vi "SUMMER SUNDAY BYTE.vi"() -> ()   [LabVIEW 2009]
uses:
  <vilib>/ULx/Create Channel.llb/ULx Create Channel (AI-Voltage-Basic).vi
  <vilib>/ULx/Read.llb/ULx Read (Analog DBL 1Chan 1Samp).vi
panel:
  in  "BitValue":bool
  out "POWER":bool
  out "data":dbl format="%_6g"
  out "xray":bool caption="BitValue"
  out "ENERGY LEVEL":dbl(knob) scale=0.0..15.0
  out "x*y":dbl
  out "Beam Pot":dbl format="%_6g"
  out "READY 2":bool
  out "DUMP":bool
  out "POWER":bool
  out "?":bool
  out "?":bool
  out "?":bool
  out "?":bool
  out "?":bool
  out "?":bool
  out "?":bool
  out "?":bool
  out "?":bool
  out "?":bool
  out "OPEN":bool
  out "CLOSED":bool
  in  "READY":bool
  out "FAULT":bool
  out "MAGNET FORCE":dbl(slide) scale=0.0..10.0
  out "READY":bool
  out "TEMPERATURE":dbl(slide) scale=0.0..10.0
  in  "stop":bool
  out "?":bool
  out "?":bool
  out "?":bool
  out "?":bool
  in  "FAULT":bool
  out "POWER":bool
  out "FLOW IN GPM":dbl(knob) scale=0.0..15.0
  # "USERS LAB AREA"
  # "BEAM STATUS"
  # "ROOM"
  # "XRAY"
  # "PUMP STATION"
  # "MAGNET STATUS"
  # "ORBIT"
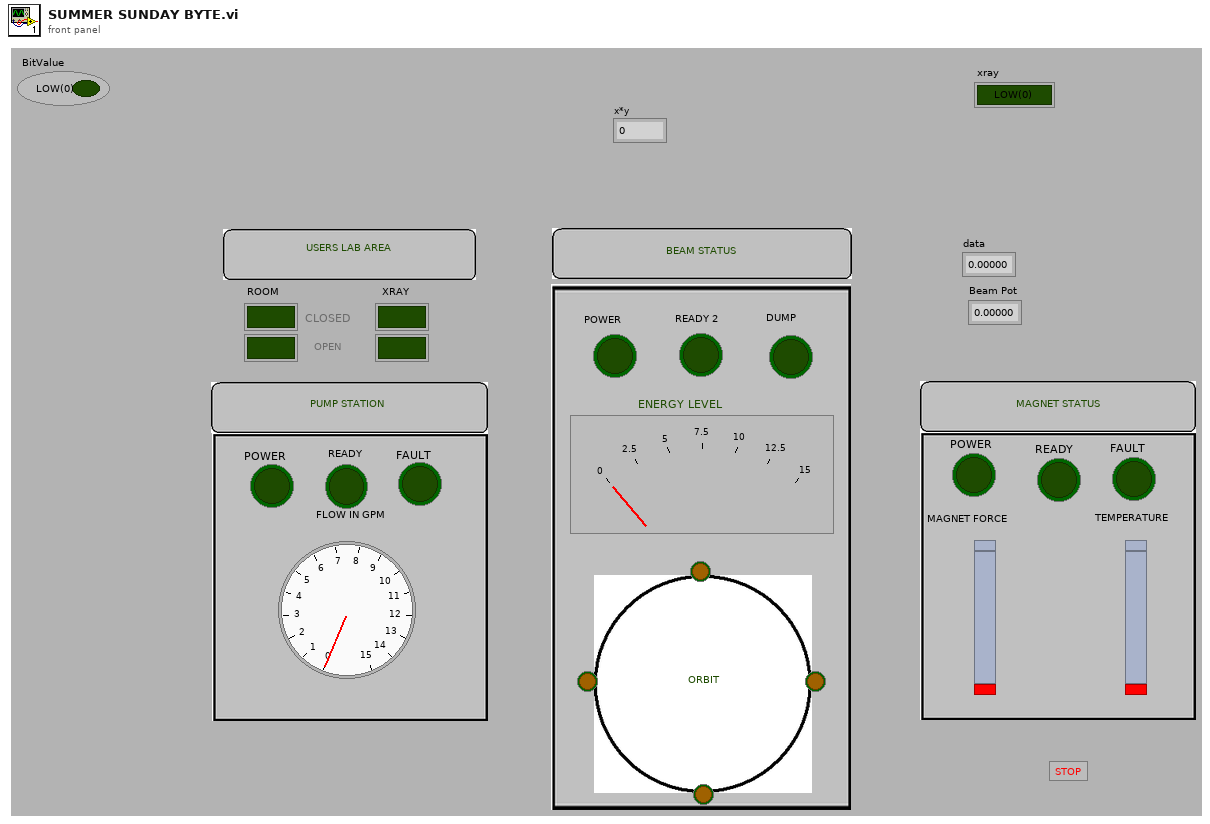
[diagram p1: front panel]
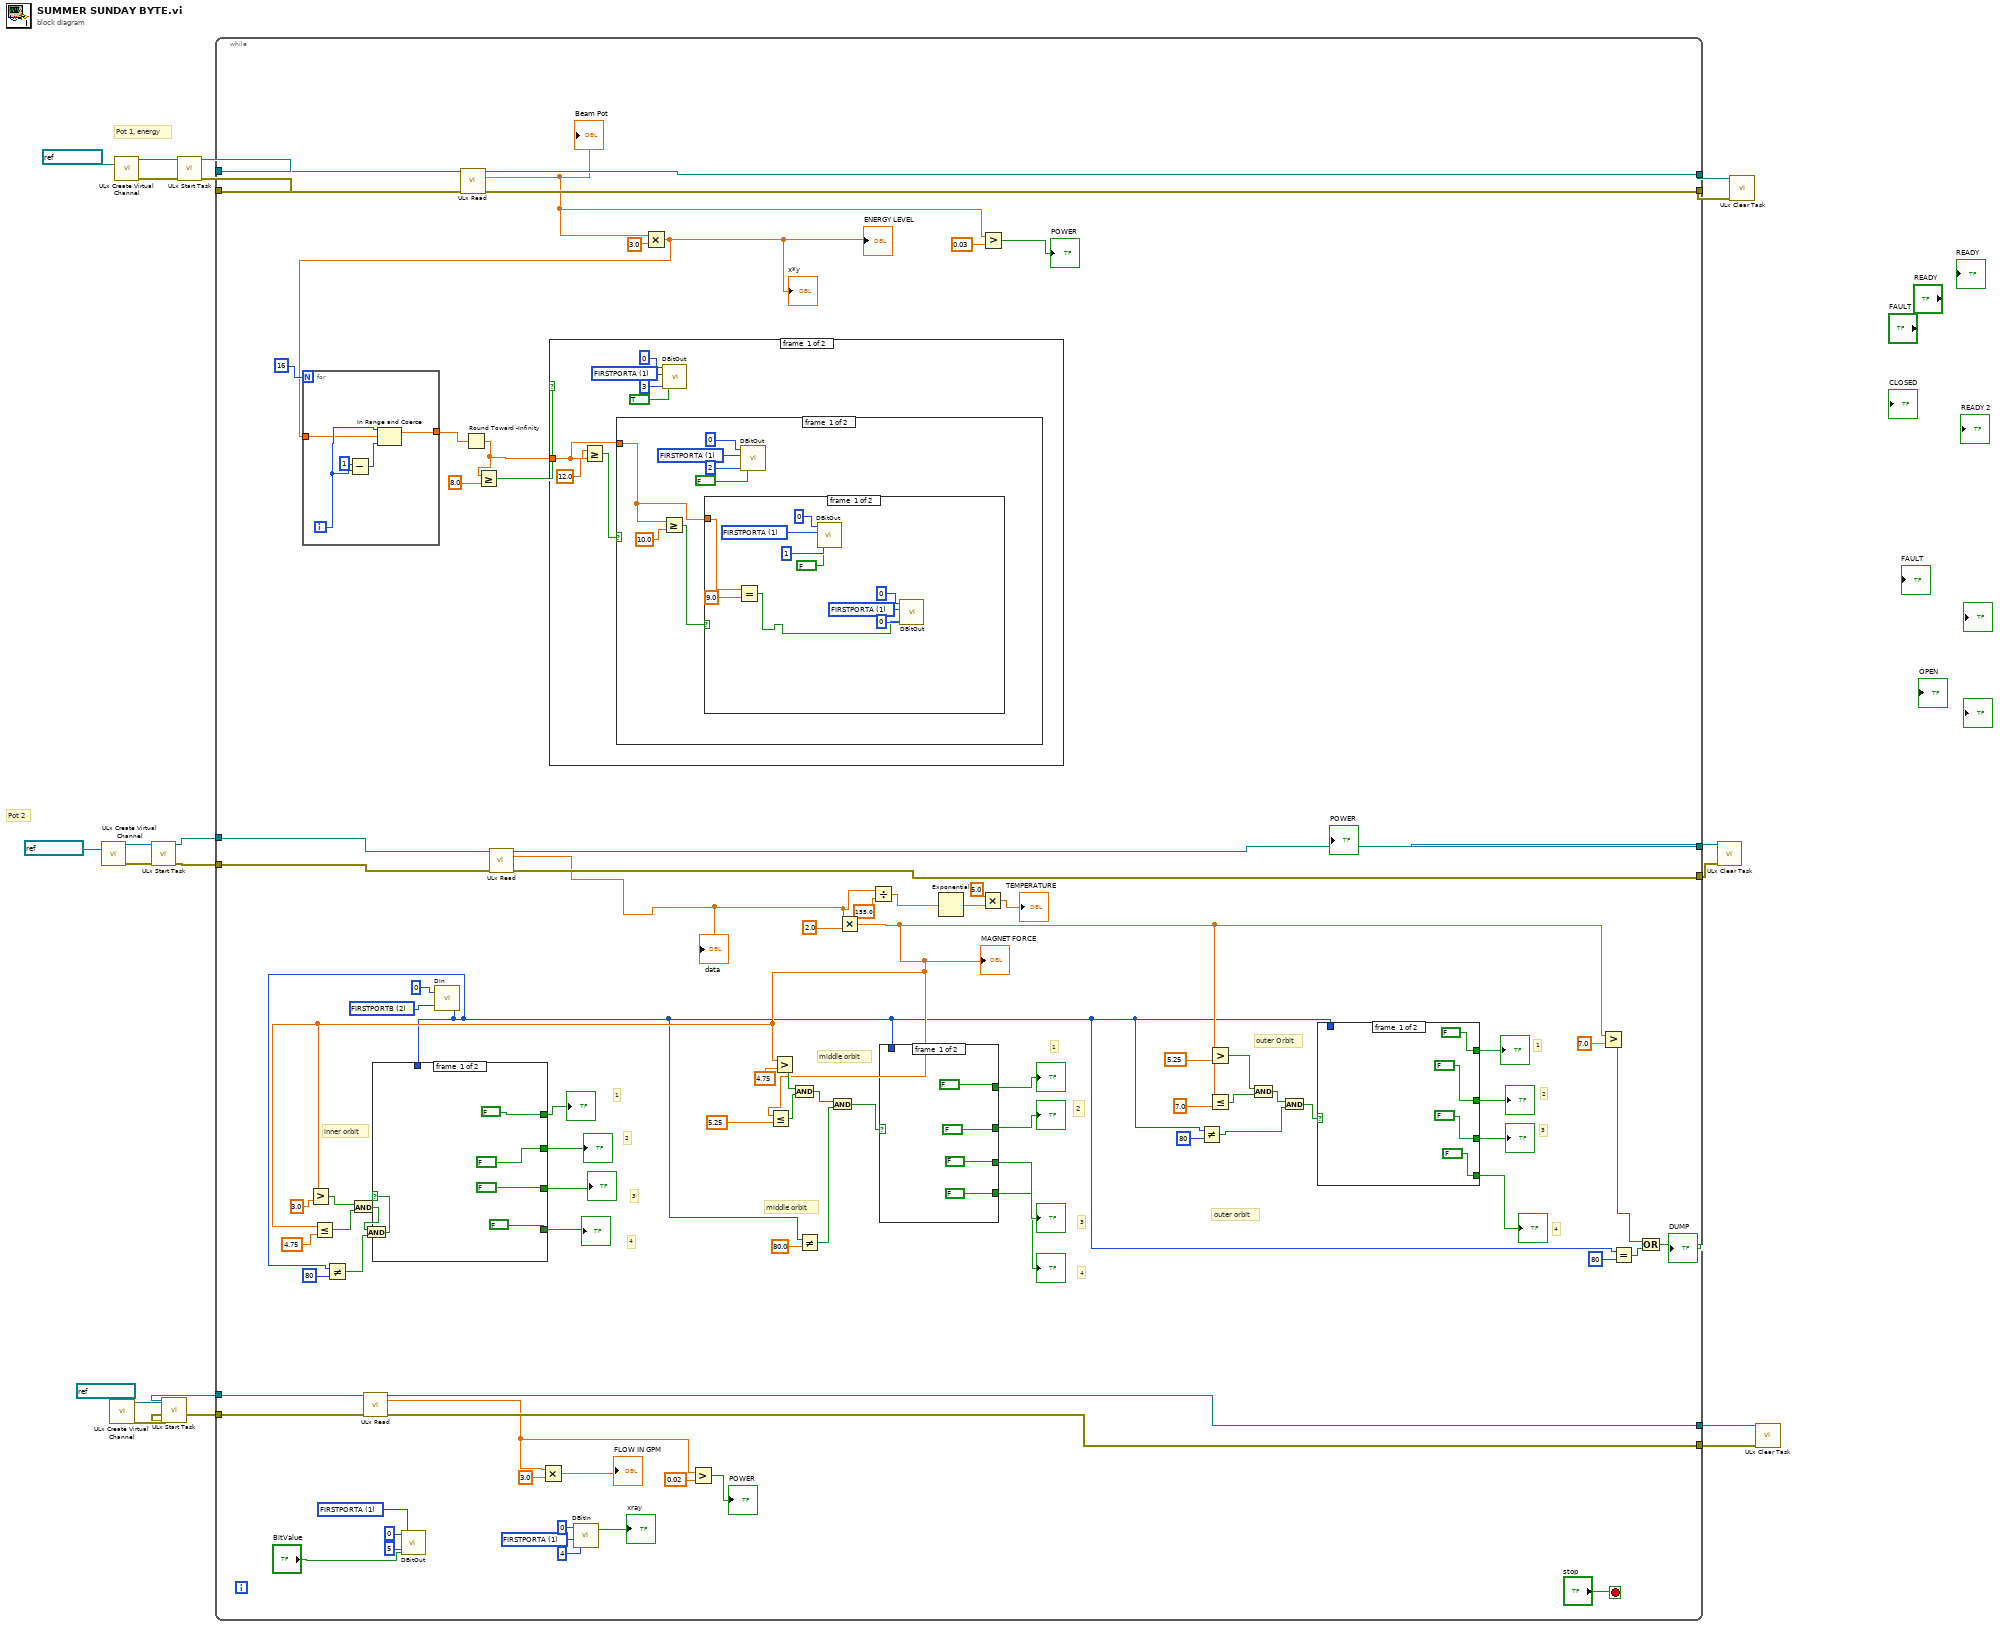
[diagram p0: block diagram]
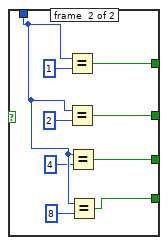
[diagram p2: hidden frame]
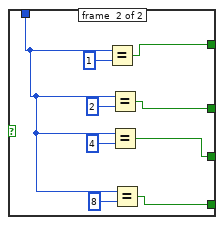
[diagram p3: hidden frame]
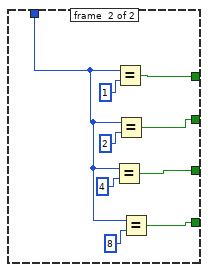
[diagram p4: hidden frame]
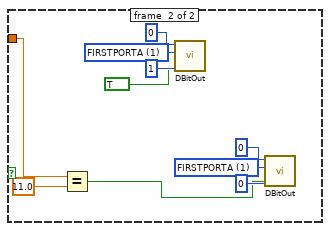
[diagram p5: hidden frame]
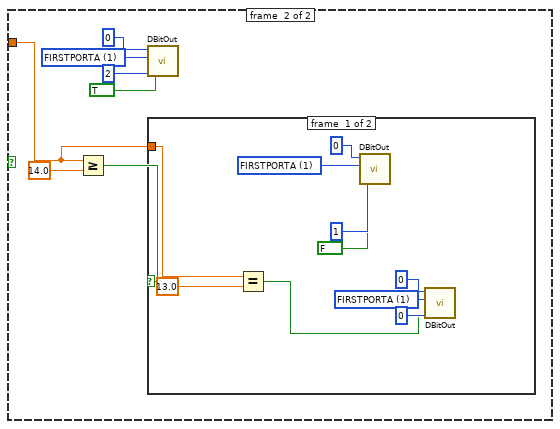
[diagram p6: hidden frame]
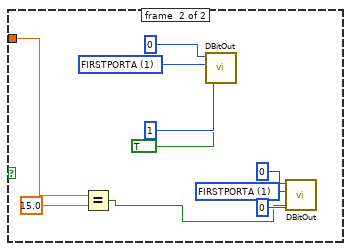
[diagram p7: hidden frame]
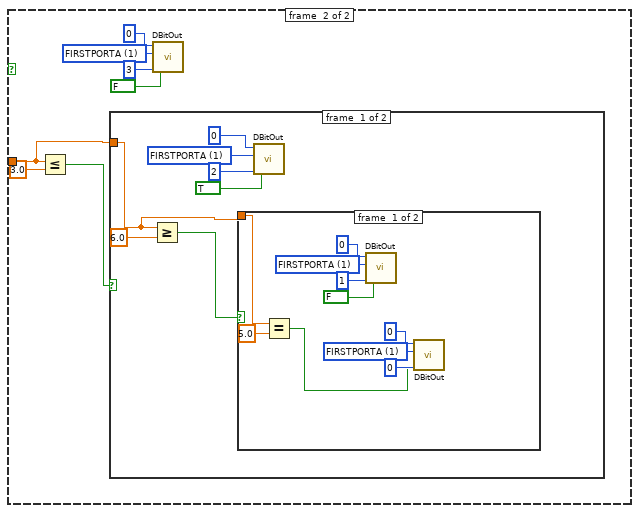
[diagram p8: hidden frame]
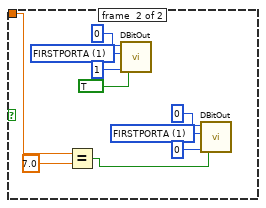
[diagram p9: hidden frame]
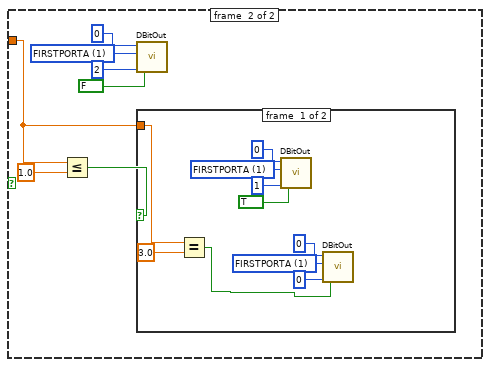
[diagram p10: hidden frame]
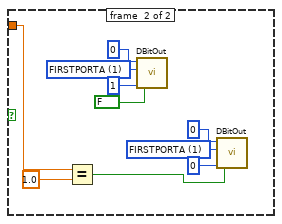
[diagram p11: hidden frame]
diagram:
  # "Pot 2"
  # "Pot 1, energy"
  n1 = call-poly <vilib>:"ULx Create Virtual Channel.vi"("physical channels"=refnum<k21> "Dev0/Ai1") -> ("task out"=w15:refnum<k24>, "error out"=w14:errorcluster)  [unwired: 13 in]
  n2 = call-poly <vilib>:"ULx Create Virtual Channel.vi"("physical channels"=refnum<k21> "Dev0/Ai2") -> ("task out"=w7:refnum<k24>, "error out"=w6:errorcluster)  [unwired: 13 in]
  n3 = call-poly <vilib>:"ULx Create Virtual Channel.vi"("physical channels"=refnum<k21> "Dev0/Ai0") -> ("task out"=w21:refnum<k24>, "error out"=w20:errorcluster)  [unwired: 13 in]
  n4 = call <vilib>:"ULx Start Task.vi"("task in"=w15, "error in"=w14) -> ("task out"=w13:refnum<k24>, "error out"=w12:errorcluster)  [unwired: 12 in]
  n5 = call <vilib>:"ULx Start Task.vi"("task in"=w7, "error in"=w6) -> ("task out"=w5:refnum<k24>, "error out"=w4:errorcluster)  [unwired: 12 in]
  n6 = call <vilib>:"ULx Start Task.vi"("task in"=w21, "error in"=w20) -> ("task out"=w19:refnum<k24>, "error out"=w18:errorcluster)  [unwired: 12 in]
  n7 = while {
    tunnel: w19 -> [w108]
    tunnel: w18 -> [w107]
    tunnel: [w106] -> w17
    tunnel: [w105] -> w16
    tunnel: w13 -> [w97]
    tunnel: w12 -> [w96]
    tunnel: [w95] -> w11
    tunnel: [w94] -> w10
    tunnel: w5 -> [w42]
    tunnel: w4 -> [w41]
    tunnel: [w40] -> w2
    tunnel: [w39] -> w1
    stop <- "stop" stop-if-true
    w34 = 1 items=["AUXPORT", "FIRSTPORTA"] ("PortType")
    w37 = u32 1 items=["AUXPORT", "FIRSTPORTA"] ("PortType")
    w68 = 2 items=["AUXPORT", "FIRSTPORTA", "FIRSTPORTB", "FIRSTPORTCL", "FIRSTPORTCH", "SECONDPORTA", "SECONDPORTB", "SECONDPORTCL", "SECONDPORTCH", "THIRDPORTA", "THIRDPORTB", "THIRDPORTCL", "THIRDPORTCH", "FOURTHPORTA", "FOURTHPORTB", "FOURTHPORTCL", "FOURTHPORTCH", "FIFTHPORTA", "FIFTHPORTB", "FIFTHPORTCL", "FIFTHPORTCH", "SIXTHPORTA", "SIXTHPORTB", "SIXTHPORTCL", "SIXTHPORTCH", "SEVENTHPORTA", "SEVENTHPORTB", "SEVENTHPORTCL", "SEVENTHPORTCH", "EIGTHPORTA", "EIGHTHPORTB", "EIGHTHPORTCL", "EIGHTHPORTCH"] ("PortNum")
    # "outer Orbit"
    # "middle orbit"
    # "4"
    # "3"
    # "2"
    # "1"
    # "1"
    # "2"
    # "3"
    # "4"
    # "4"
    # "3"
    # "2"
    # "1"
    # "outer orbit"
    # "inner orbit"
    # "middle orbit"
    n8 = call-poly <vilib>:"ULx Read.vi"("task in"=w42, "error in"=w41) -> ("task out"=w40:refnum<k24>, "data"=w28:dbl, "error out"=w39:errorcluster)  [unwired: 11 in]
    n9 = call <menus>:"DBitOut.VI"("BitValue"="BitValue", "BitNum"=u32 5, "PortType"=w37, "BoardNum"=u32 0) -> ()  [unwired: 1 out]
    n10 = call <menus>:"DIn.VI"("PortNum"=w68, "BoardNum"=u32 0) -> ("DataValue"=w54:i16)  [unwired: 1 out]
    n11 = Not Equal?(x=w54, y=i16 80) -> (x != y?=w80:bool)
    n12 = call-poly <vilib>:"ULx Read.vi"("task in"=w108, "error in"=w107) -> ("task out"=w106:refnum<k24>, "data"=w25:dbl, "error out"=w105:errorcluster)  [unwired: 11 in]
    "Beam Pot" <- w25
    n13 = call-poly <vilib>:"ULx Read.vi"("task in"=w97, "error in"=w96) -> ("task out"=w95:refnum<k24>, "data"=w23:dbl, "error out"=w94:errorcluster)  [unwired: 11 in]
    "data" <- w23
    n14 = Multiply(x=w28, y=3.0) -> (x*y=→"FLOW IN GPM":dbl)
    n15 = call <menus>:"DBitIn.VI"("BitNum"=4, "PortType"=w34, "BoardNum"=u32 0) -> ("BitValue"=→"xray":bool)  [unwired: 1 out]
    n16 = Multiply(x=w25, y=3.0) -> (x*y=w98:dbl)
    "x*y" <- w98
    "ENERGY LEVEL" <- w98
    n17 = for {
      N: 16 -> [_]
      tunnel: w98 -> [w272]
      tunnel: [w271] -> w102
      i -> [w274]
      n18 = Subtract(x=1, y=w274) -> (x-y=w275:i32)
      n19 = In Range and Coerce(upper limit=w274, x=w272, lower limit=w275) -> (coerced(x)=w271:dbl)  [unwired: 1 out]
    }
    n20 = Round Toward -Infinity(1:w102) -> (0:w99:dbl)
    n21 = Greater Or Equal?(x=w99, y=8.0) -> (x >= y?=w100:bool)
    n22 = case shown="False" w100 {
      tunnel: w99 -> [w149 w210]
      frame #0 {
        w154 = u32 1 items=["AUXPORT", "FIRSTPORTA"] ("PortType")
        n23 = Greater Or Equal?(x=w149, y=12.0) -> (x >= y?=w150:bool)
        n24 = case shown="True" w150 {
          tunnel: w149 -> [w156 w183]
          frame #0 {
            w161 = u32 1 items=["AUXPORT", "FIRSTPORTA"] ("PortType")
            n25 = Greater Or Equal?(x=w156, y=10.0) -> (x >= y?=w157:bool)
            n26 = case shown="True" w157 {
              tunnel: w156 -> [w168 w179]
              frame #0 {
                w166 = u32 1 items=["AUXPORT", "FIRSTPORTA"] ("PortType")
                w171 = u32 1 items=["AUXPORT", "FIRSTPORTA"] ("PortType")
                n27 = Equal?(x=w168, y=9.0) -> (x = y?=w163:bool)
                n28 = call <menus>:"DBitOut.VI"("BitValue"=FALSE, "BitNum"=u32 1, "PortType"=w171, "BoardNum"=u32 0) -> ()  [unwired: 1 out]
                n29 = call <menus>:"DBitOut.VI"("BitValue"=w163, "BitNum"=u32 0, "PortType"=w166, "BoardNum"=u32 0) -> ()  [unwired: 1 out]
              }
              frame #1 {
                w176 = u32 1 items=["AUXPORT", "FIRSTPORTA"] ("PortType")
                w181 = u32 1 items=["AUXPORT", "FIRSTPORTA"] ("PortType")
                n30 = Equal?(x=w179, y=11.0) -> (x = y?=w173:bool)
                n31 = call <menus>:"DBitOut.VI"("BitValue"=TRUE, "BitNum"=u32 1, "PortType"=w181, "BoardNum"=u32 0) -> ()  [unwired: 1 out]
                n32 = call <menus>:"DBitOut.VI"("BitValue"=w173, "BitNum"=u32 0, "PortType"=w176, "BoardNum"=u32 0) -> ()  [unwired: 1 out]
              }
            }
            n33 = call <menus>:"DBitOut.VI"("BitValue"=FALSE, "BitNum"=u32 2, "PortType"=w161, "BoardNum"=u32 0) -> ()  [unwired: 1 out]
          }
          frame #1 {
            w188 = u32 1 items=["AUXPORT", "FIRSTPORTA"] ("PortType")
            n34 = Greater Or Equal?(x=w183, y=14.0) -> (x >= y?=w184:bool)
            n35 = call <menus>:"DBitOut.VI"("BitValue"=TRUE, "BitNum"=u32 2, "PortType"=w188, "BoardNum"=u32 0) -> ()  [unwired: 1 out]
            n36 = case shown="False" w184 {
              tunnel: w183 -> [w195 w205]
              frame #0 {
                w193 = u32 1 items=["AUXPORT", "FIRSTPORTA"] ("PortType")
                w198 = u32 1 items=["AUXPORT", "FIRSTPORTA"] ("PortType")
                n37 = Equal?(x=w195, y=13.0) -> (x = y?=w190:bool)
                n38 = call <menus>:"DBitOut.VI"("BitValue"=FALSE, "BitNum"=u32 1, "PortType"=w198, "BoardNum"=u32 0) -> ()  [unwired: 1 out]
                n39 = call <menus>:"DBitOut.VI"("BitValue"=w190, "BitNum"=u32 0, "PortType"=w193, "BoardNum"=u32 0) -> ()  [unwired: 1 out]
              }
              frame #1 {
                w203 = u32 1 items=["AUXPORT", "FIRSTPORTA"] ("PortType")
                w208 = u32 1 items=["AUXPORT", "FIRSTPORTA"] ("PortType")
                n40 = Equal?(x=w205, y=15.0) -> (x = y?=w200:bool)
                n41 = call <menus>:"DBitOut.VI"("BitValue"=TRUE, "BitNum"=u32 1, "PortType"=w208, "BoardNum"=u32 0) -> ()  [unwired: 1 out]
                n42 = call <menus>:"DBitOut.VI"("BitValue"=w200, "BitNum"=u32 0, "PortType"=w203, "BoardNum"=u32 0) -> ()  [unwired: 1 out]
              }
            }
          }
        }
        n43 = call <menus>:"DBitOut.VI"("BitValue"=TRUE, "BitNum"=u32 3, "PortType"=w154, "BoardNum"=u32 0) -> ()  [unwired: 1 out]
      }
      frame #1 {
        w215 = u32 1 items=["AUXPORT", "FIRSTPORTA"] ("PortType")
        n44 = Less Or Equal?(x=w210, y=3.0) -> (x <= y?=w211:bool)
        n45 = case shown="False" w211 {
          tunnel: w210 -> [w217 w244]
          frame #0 {
            w222 = u32 1 items=["AUXPORT", "FIRSTPORTA"] ("PortType")
            n46 = Greater Or Equal?(x=w217, y=6.0) -> (x >= y?=w218:bool)
            n47 = case shown="False" w218 {
              tunnel: w217 -> [w226 w239]
              frame #0 {
                w228 = u32 1 items=["AUXPORT", "FIRSTPORTA"] ("PortType")
                w232 = u32 1 items=["AUXPORT", "FIRSTPORTA"] ("PortType")
                n48 = Equal?(x=w226, y=5.0) -> (x = y?=w224:bool)
                n49 = call <menus>:"DBitOut.VI"("BitValue"=FALSE, "BitNum"=u32 1, "PortType"=w232, "BoardNum"=u32 0) -> ()  [unwired: 1 out]
                n50 = call <menus>:"DBitOut.VI"("BitValue"=w224, "BitNum"=u32 0, "PortType"=w228, "BoardNum"=u32 0) -> ()  [unwired: 1 out]
              }
              frame #1 {
                w236 = u32 1 items=["AUXPORT", "FIRSTPORTA"] ("PortType")
                w242 = u32 1 items=["AUXPORT", "FIRSTPORTA"] ("PortType")
                n51 = Equal?(x=w239, y=7.0) -> (x = y?=w234:bool)
                n52 = call <menus>:"DBitOut.VI"("BitValue"=TRUE, "BitNum"=u32 1, "PortType"=w242, "BoardNum"=u32 0) -> ()  [unwired: 1 out]
                n53 = call <menus>:"DBitOut.VI"("BitValue"=w234, "BitNum"=u32 0, "PortType"=w236, "BoardNum"=u32 0) -> ()  [unwired: 1 out]
              }
            }
            n54 = call <menus>:"DBitOut.VI"("BitValue"=TRUE, "BitNum"=u32 2, "PortType"=w222, "BoardNum"=u32 0) -> ()  [unwired: 1 out]
          }
          frame #1 {
            w249 = u32 1 items=["AUXPORT", "FIRSTPORTA"] ("PortType")
            n55 = Less Or Equal?(x=w244, y=1.0) -> (x <= y?=w245:bool)
            n56 = call <menus>:"DBitOut.VI"("BitValue"=FALSE, "BitNum"=u32 2, "PortType"=w249, "BoardNum"=u32 0) -> ()  [unwired: 1 out]
            n57 = case shown="True" w245 {
              tunnel: w244 -> [w256 w266]
              frame #0 {
                w253 = u32 1 items=["AUXPORT", "FIRSTPORTA"] ("PortType")
                w259 = u32 1 items=["AUXPORT", "FIRSTPORTA"] ("PortType")
                n58 = Equal?(x=w256, y=3.0) -> (x = y?=w251:bool)
                n59 = call <menus>:"DBitOut.VI"("BitValue"=TRUE, "BitNum"=u32 1, "PortType"=w259, "BoardNum"=u32 0) -> ()  [unwired: 1 out]
                n60 = call <menus>:"DBitOut.VI"("BitValue"=w251, "BitNum"=u32 0, "PortType"=w253, "BoardNum"=u32 0) -> ()  [unwired: 1 out]
              }
              frame #1 {
                w263 = u32 1 items=["AUXPORT", "FIRSTPORTA"] ("PortType")
                w269 = u32 1 items=["AUXPORT", "FIRSTPORTA"] ("PortType")
                n61 = Equal?(x=w266, y=1.0) -> (x = y?=w261:bool)
                n62 = call <menus>:"DBitOut.VI"("BitValue"=FALSE, "BitNum"=u32 1, "PortType"=w269, "BoardNum"=u32 0) -> ()  [unwired: 1 out]
                n63 = call <menus>:"DBitOut.VI"("BitValue"=w261, "BitNum"=u32 0, "PortType"=w263, "BoardNum"=u32 0) -> ()  [unwired: 1 out]
              }
            }
          }
        }
        n64 = call <menus>:"DBitOut.VI"("BitValue"=FALSE, "BitNum"=u32 3, "PortType"=w215, "BoardNum"=u32 0) -> ()  [unwired: 1 out]
      }
    }
    n65 = Greater?(x=w28, y=0.02) -> (0:→"POWER":bool)
    n66 = Not Equal?(x=w54, y=80.0) -> (x != y?=w64:bool)
    n67 = Multiply(x=w23, y=2.0) -> (x*y=w73:dbl)
    "MAGNET FORCE" <- w73
    n68 = Greater?(x=w73, y=3.0) -> (0:w90:bool)
    n69 = Less Or Equal?(x=w73, y=4.75) -> (x <= y?=w91:bool)
    n70 = And(x=w90, y=w91) -> (x .and. y?=w82:bool)
    n71 = And(x=w82, y=w80) -> (x .and. y?=w81:bool)
    n72 = case shown="True" w81 {
      tunnel: [FALSE w143] -> w50
      tunnel: [FALSE w142] -> w51
      tunnel: [FALSE w141] -> w48
      tunnel: [FALSE w140] -> w49
      tunnel: w54 -> [_ w148]
      frame #0 {
      }
      frame #1 {
        n73 = Equal?(x=w148, y=i16 4) -> (x = y?=w141:bool)
        n74 = Equal?(x=w148, y=i16 1) -> (x = y?=w143:bool)
        n75 = Equal?(x=w148, y=i16 2) -> (x = y?=w142:bool)
        n76 = Equal?(x=w148, y=i16 8) -> (x = y?=w140:bool)
      }
    }
    "?" <- w51
    "?" <- w48
    "?" <- w49
    "?" <- w50
    n77 = Less Or Equal?(x=w73, y=5.25) -> (x <= y?=w87:bool)
    n78 = Greater?(x=w73, y=4.75) -> (0:w88:bool)
    n79 = And(x=w88, y=w87) -> (x .and. y?=w79:bool)
    n80 = And(x=w79, y=w64) -> (x .and. y?=w62:bool)
    n81 = Divide(x=w23, y=155.0) -> (x/y=w46:dbl)
    n82 = case shown="False" w62 {
      tunnel: [FALSE w122] -> w61
      tunnel: [FALSE w121] -> w60
      tunnel: [FALSE w120] -> w59
      tunnel: [FALSE w119] -> w58
      tunnel: w54 -> [_ w118]
      frame #0 {
      }
      frame #1 {
        n83 = Equal?(x=w118, y=i16 1) -> (x = y?=w122:bool)
        n84 = Equal?(x=w118, y=i16 2) -> (x = y?=w121:bool)
        n85 = Equal?(x=w118, y=i16 4) -> (x = y?=w120:bool)
        n86 = Equal?(x=w118, y=i16 8) -> (x = y?=w119:bool)
      }
    }
    "?" <- w61
    "?" <- w60
    "?" <- w59
    "?" <- w58
    n87 = Exponential(1:w46) -> (0:w45:dbl)
    n88 = Multiply(x=5.0, y=w45) -> (x*y=→"TEMPERATURE":dbl)
    n89 = Greater?(x=w25, y=0.03) -> (0:→"POWER":bool)
    n90 = Not Equal?(x=w54, y=i16 80) -> (x != y?=w56:bool)
    n91 = Greater?(x=w73, y=5.25) -> (0:w85:bool)
    n92 = Less Or Equal?(x=w73, y=7.0) -> (x <= y?=w84:bool)
    n93 = And(x=w85, y=w84) -> (x .and. y?=w71:bool)
    n94 = And(x=w71, y=w56) -> (x .and. y?=w70:bool)
    n95 = case shown="True" w70 {
      tunnel: [FALSE w127] -> w77
      tunnel: [FALSE w128] -> w76
      tunnel: [FALSE w129] -> w75
      tunnel: [FALSE w130] -> w74
      tunnel: w54 -> [_ w135]
      frame #0 {
      }
      frame #1 {
        n96 = Equal?(x=w135, y=i16 1) -> (x = y?=w130:bool)
        n97 = Equal?(x=w135, y=i16 2) -> (x = y?=w129:bool)
        n98 = Equal?(x=w135, y=i16 4) -> (x = y?=w128:bool)
        n99 = Equal?(x=w135, y=i16 8) -> (x = y?=w127:bool)
      }
    }
    "?" <- w74
    "?" <- w75
    "?" <- w76
    "?" <- w77
    n100 = Greater?(x=w73, y=7.0) -> (0:w72:bool)
    n101 = Equal?(x=w54, y=i16 80) -> (x = y?=w52:bool)
    n102 = Or(x=w72, y=w52) -> (x .or. y?=→"DUMP":bool)
  }
  n103 = call <vilib>:"ULx Clear Task.vi"("task in"=w11, "error in"=w10) -> ()  [unwired: 13 in, 1 out]
  n104 = call <vilib>:"ULx Clear Task.vi"("task in"=w17, "error in"=w16) -> ()  [unwired: 13 in, 1 out]
  n105 = call <vilib>:"ULx Clear Task.vi"("task in"=w2, "error in"=w1) -> ()  [unwired: 13 in, 1 out]
